vi "VL Type.vi"(8 "error in (no error)":errorcluster, 11 "Scale in":refnum<class "Scale.lvclass">) -> (0 "error out":errorcluster, 2 "VL Type":T1, 3 "Scale out":refnum<class "Scale.lvclass">)   [LabVIEW 2020, in "VolatusConfig.lvlib" / "Scale.lvclass"]
uses:
  Scale.lvclass
  Meta Type.ctl
  VolatusConfig.lvlib
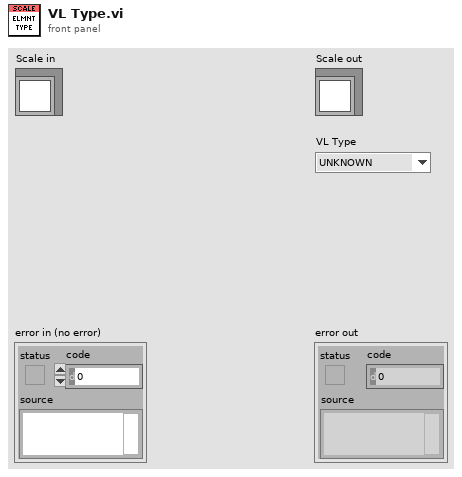
[diagram p1: front panel]
types:
  T1 = typedef "VolatusConfig.lvlib/Meta Type.ctl" = enum16{"UNKNOWN", "VL_System", "VL_Cluster", "VL_Node", "VL_Task", "VL_Group", "VL_Channel", "VL_Task_List", "VL_Scaling", "VL_Sensor", "VL_Sensor_List", "VL_Scale"}
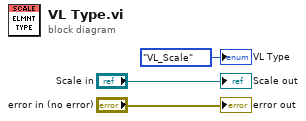
[diagram p0: block diagram]
diagram:
  "error out" <- "error in (no error)"
  "Scale out" <- "Scale in"
  "VL Type" <- Meta_Type."VL_Scale" ("VL Type")
